vi "Unpack Notification Msg.vi"(11 "Notification Msg in":refnum<class "Notification Msg.lvclass">) -> (1 "Publication Time":timestamp, 2 "Value":variant, 3 "Topic Name":string)   [LabVIEW 2015, in "Transport.lvlib" / "Notification Msg.lvclass"]
doc: "<License>\nCopyright © 2017 Composed Systems, LLC | All rights reserved\nwww.composed.io\n\nAuthor: Ethan Stern <ethan.stern@composed.io>\n\nThis software is provided \"AS IS\" WITHOUT WARRANTIES, either express or implied, AND IS FOR EDUCATIONAL PURPOSES ONLY.\n</License>"
uses:
  Notification Msg.lvclass
  Notification Msg.lvclass/Notification Msg.ctl
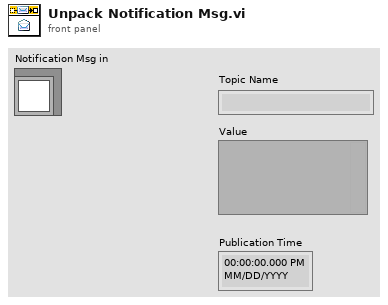
[diagram p1: front panel]
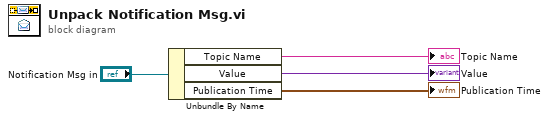
[diagram p0: block diagram]
diagram:
  n1 = Unbundle By Name("Notification Msg in") -> ("Topic Name"=→"Topic Name":string, "Value"=→"Value":variant, "Publication Time"=→"Publication Time":timestamp)
